vi "grSimTestParametersView.vi"(8 "error in (no error)":errorcluster, 9 "Cluster":T1, 10 "grSimTestEnum":T2=enum."VelocityPlanning", 11 "Parameters in":refnum<class "Parameters.lvclass">) -> (0 "error out":errorcluster, 3 "Parameters out":refnum<class "Parameters.lvclass">)   [LabVIEW 2020, in "Parameters.lvclass"]
uses:
  Parameters.lvclass
  Game_class/VelocityPlanningTest/Controls/testMode.ctl
  GrsimTestRef.ctl
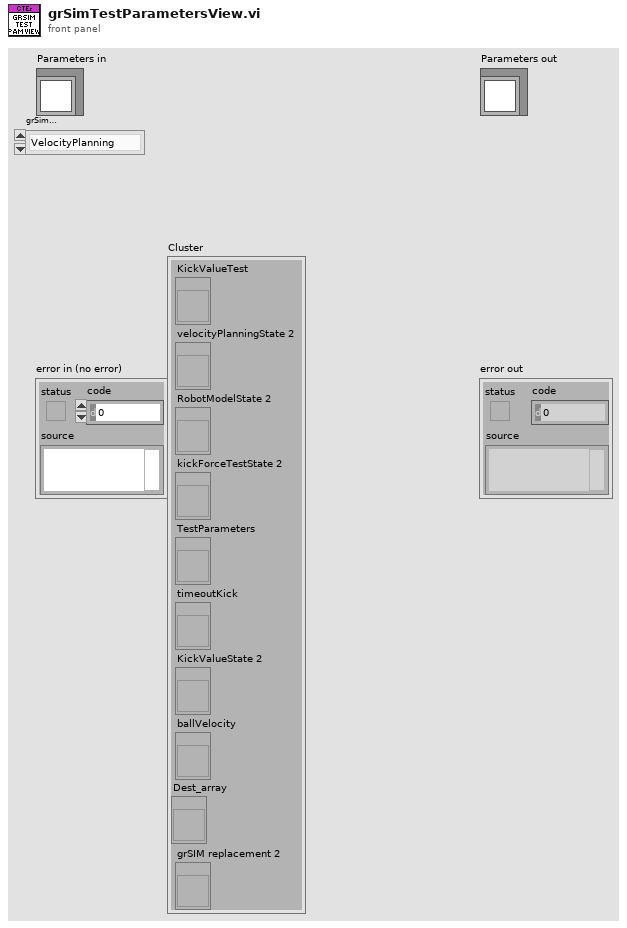
[diagram p1: front panel]
types:
  T1 = typedef "GrsimTestRef.ctl" = cluster{"KickValueTest":refnum<vi>, "velocityPlanningState 2":refnum<vi>, "RobotModelState 2":refnum<vi>, "kickForceTestState 2":refnum<vi>, "TestParameters":refnum<vi>, "timeoutKick":refnum<vi>, "KickValueState 2":refnum<vi>, "ballVelocity":refnum<vi>, "grSIM replacement 2":refnum<vi>, "Dest_array":refnum<vi>}
  T2 = typedef "testMode.ctl" = enum16{"KickForce", "KickValue", "VelocityPlanning", "RobotModel"}
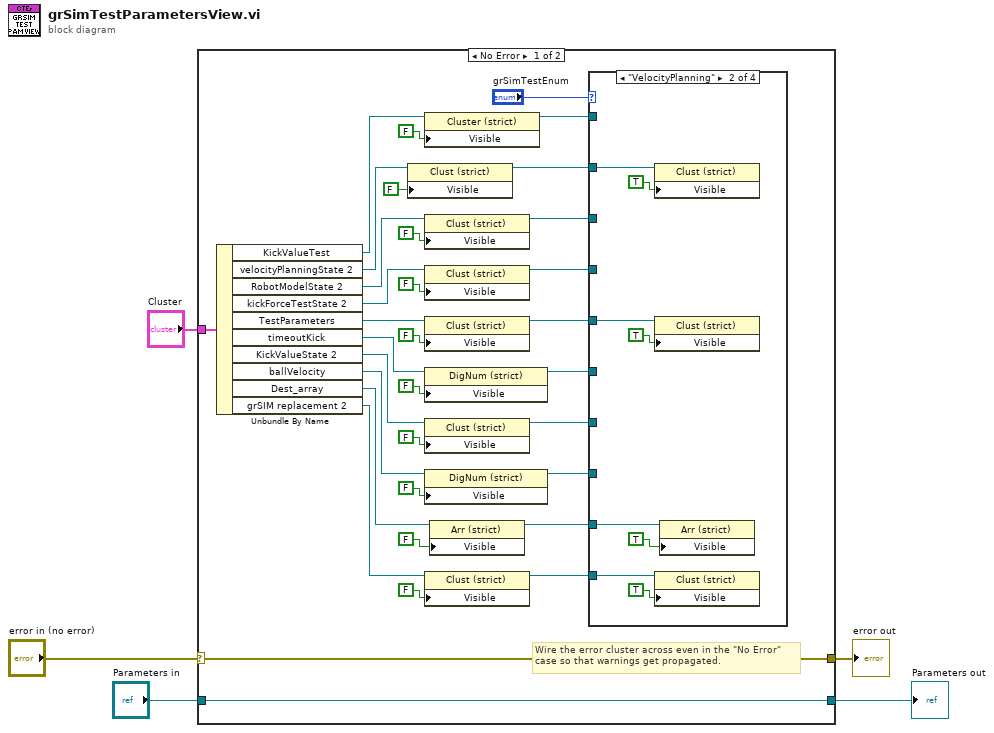
[diagram p0: block diagram]
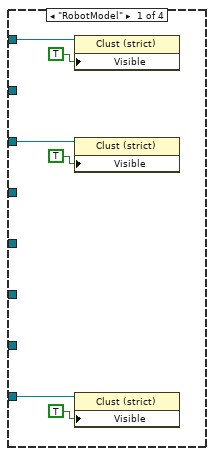
[diagram p2: hidden frame]
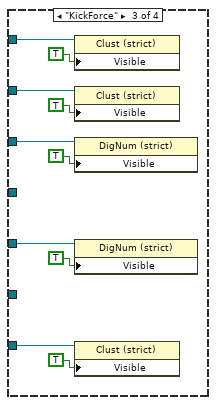
[diagram p3: hidden frame]
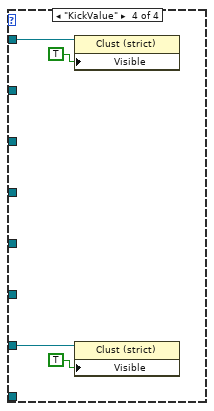
[diagram p4: hidden frame]
diagram:
  n1 = case shown="No Error" "error in (no error)" {
    selector: "error in (no error)" -> [w38 w69]
    tunnel: [w38 w69] -> w4
    tunnel: [w39 w68] -> w2
    tunnel: "Parameters in" -> [w39 w68]
    tunnel: "Cluster" -> [w34 _]
    frame No Error {
      # "Wire the error cluster across even in the \"No Error\"\ncase so that warnings get propagated."
      n2 = Unbundle By Name(w34) -> ("KickValueTest"=w33:refnum<vi>, "velocityPlanningState 2"=w15:refnum<vi>, "RobotModelState 2"=w16:refnum<vi>, "kickForceTestState 2"=w23:refnum<vi>, "TestParameters"=w22:refnum<vi>, "timeoutKick"=w21:refnum<vi>, "KickValueState 2"=w20:refnum<vi>, "ballVelocity"=w19:refnum<vi>, "Dest_array"=w18:refnum<vi>, "grSIM replacement 2"=w17:refnum<vi>)
      n3 = property on="Property Node" class="Clust (strict)"(reference=w15, "Visible"=FALSE) -> (reference out=w14:refnum<vi>)  [unwired: 1 in, 1 out]
      n4 = property on="Property Node" class="Cluster (strict)"(reference=w33, "Visible"=FALSE) -> (reference out=w36:refnum<vi>)  [unwired: 1 in, 1 out]
      n5 = property on="Property Node" class="Clust (strict)"(reference=w16, "Visible"=FALSE) -> (reference out=w31:refnum<vi>)  [unwired: 1 in, 1 out]
      n6 = property on="Property Node" class="Clust (strict)"(reference=w23, "Visible"=FALSE) -> (reference out=w13:refnum<vi>)  [unwired: 1 in, 1 out]
      n7 = property on="Property Node" class="Clust (strict)"(reference=w22, "Visible"=FALSE) -> (reference out=w12:refnum<vi>)  [unwired: 1 in, 1 out]
      n8 = property on="Property Node" class="DigNum (strict)"(reference=w21, "Visible"=FALSE) -> (reference out=w11:refnum<vi>)  [unwired: 1 in, 1 out]
      n9 = property on="Property Node" class="Clust (strict)"(reference=w20, "Visible"=FALSE) -> (reference out=w10:refnum<vi>)  [unwired: 1 in, 1 out]
      n10 = property on="Property Node" class="DigNum (strict)"(reference=w19, "Visible"=FALSE) -> (reference out=w9:refnum<vi>)  [unwired: 1 in, 1 out]
      n11 = property on="Property Node" class="Clust (strict)"(reference=w17, "Visible"=FALSE) -> (reference out=w7:refnum<vi>)  [unwired: 1 in, 1 out]
      n12 = property on="Property Node" class="Arr (strict)"(reference=w18, "Visible"=FALSE) -> (reference out=w8:refnum<vi>)  [unwired: 1 in, 1 out]
      n13 = case shown="\"VelocityPlanning\"" "grSimTestEnum" {
        tunnel: w36 -> [_ _ _ w67]
        tunnel: w31 -> [w44 _ _ _]
        tunnel: w14 -> [_ w46 _ _]
        tunnel: w13 -> [_ _ w54 _]
        tunnel: w12 -> [w41 w51 w61 _]
        tunnel: w11 -> [_ _ w57 _]
        tunnel: w10 -> [_ _ _ w65]
        tunnel: w9 -> [_ _ w56 _]
        tunnel: w8 -> [_ w47 _ _]
        tunnel: w7 -> [w40 w50 w60 _]
        frame "RobotModel" {
          n14 = property on="Property Node" class="Clust (strict)"(reference=w44, "Visible"=TRUE) -> ()  [unwired: 1 in, 2 out]
          n15 = property on="Property Node" class="Clust (strict)"(reference=w41, "Visible"=TRUE) -> ()  [unwired: 1 in, 2 out]
          n16 = property on="Property Node" class="Clust (strict)"(reference=w40, "Visible"=TRUE) -> ()  [unwired: 1 in, 2 out]
        }
        frame "VelocityPlanning" {
          n17 = property on="Property Node" class="Clust (strict)"(reference=w46, "Visible"=TRUE) -> ()  [unwired: 1 in, 2 out]
          n18 = property on="Property Node" class="Clust (strict)"(reference=w51, "Visible"=TRUE) -> ()  [unwired: 1 in, 2 out]
          n19 = property on="Property Node" class="Clust (strict)"(reference=w50, "Visible"=TRUE) -> ()  [unwired: 1 in, 2 out]
          n20 = property on="Property Node" class="Arr (strict)"(reference=w47, "Visible"=TRUE) -> ()  [unwired: 1 in, 2 out]
        }
        frame "KickForce" {
          n21 = property on="Property Node" class="Clust (strict)"(reference=w54, "Visible"=TRUE) -> ()  [unwired: 1 in, 2 out]
          n22 = property on="Property Node" class="Clust (strict)"(reference=w61, "Visible"=TRUE) -> ()  [unwired: 1 in, 2 out]
          n23 = property on="Property Node" class="DigNum (strict)"(reference=w57, "Visible"=TRUE) -> ()  [unwired: 1 in, 2 out]
          n24 = property on="Property Node" class="DigNum (strict)"(reference=w56, "Visible"=TRUE) -> ()  [unwired: 1 in, 2 out]
          n25 = property on="Property Node" class="Clust (strict)"(reference=w60, "Visible"=TRUE) -> ()  [unwired: 1 in, 2 out]
        }
        frame "KickValue" {
          n26 = property on="Property Node" class="Clust (strict)"(reference=w67, "Visible"=TRUE) -> ()  [unwired: 1 in, 2 out]
          n27 = property on="Property Node" class="Clust (strict)"(reference=w65, "Visible"=TRUE) -> ()  [unwired: 1 in, 2 out]
        }
      }
    }
    frame Error {
    }
  }
  "error out" <- w4
  "Parameters out" <- w2
